vi "Delete Temp Files.vi"(8 "error in":errorcluster, 11 "New PE Folder":path) -> (0 "error out":errorcluster)   [LabVIEW 2020, in "ADAS_IO_Template_MDO.lvclass"]
uses:
  ADAS_IO_Template_MDO.lvclass
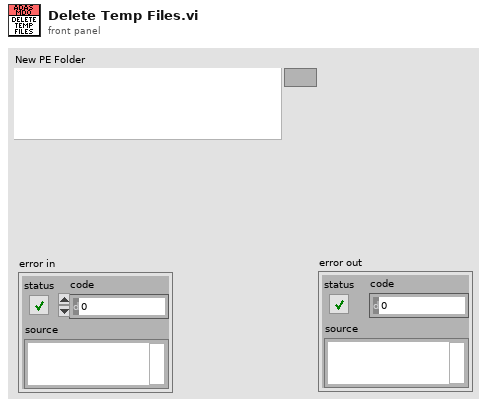
[diagram p1: front panel]
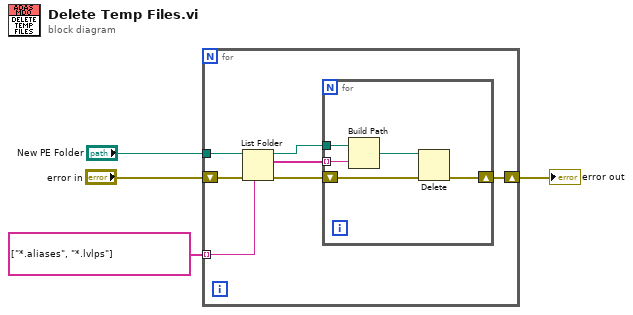
[diagram p0: block diagram]
diagram:
  n1 = for {
    tunnel: "New PE Folder" -> [w10]
    shift-right: [w6] -> w2
    shift-left: "error in" -> [w11]
    tunnel: string[] ["*.aliases", "*.lvlps"] -> [w5] mode=indexing
    n2 = List Folder(path=w10, pattern=w5, error in=w11) -> (path out=w7:path, filenames=w8:string[], error out=w9:errorcluster)  [unwired: 1 in, 1 out]
    n3 = for {
      tunnel: w8 -> [w15] mode=indexing
      shift-right: [w12] -> w6
      shift-left: w9 -> [w14]
      tunnel: w7 -> [w16]
      n4 = Build Path(base path=w16, name or relative path=w15) -> (appended path=w13:path)
      n5 = Delete(path (use dialog)=w13, error in=w14) -> (error out=w12:errorcluster)  [unwired: 3 in, 2 out]
    }
  }
  "error out" <- w2
